vi "Get Callers Cache.vi"(8 "error in (no error)":errorcluster, 11 "WorkSpace / Repo path":path) -> (0 "error out":errorcluster, 1 "LV Version Mismatched VI":path[](array[path]), 2 "Status":string, 3 "Caller Map":map{string, string[]}(c390))   [LabVIEW 2019, in "Hawkeye.lvlib"]
uses:
  Hawkeye.lvlib
  c1dc875a-4590-4514-8f55-1f0bbeb3d42e.vi
  f2e1f123-2e97-488a-9f38-c5ab8c69dbb8.vi
  3dc4041e-3bdf-4db9-bc93-15cebc6804b8.vi
  <userlib>/_OpenG.lib/array/array.llb/Search 1D Array (String)__ogtk.vi
panel:
  # "Generating Linker Cache file"
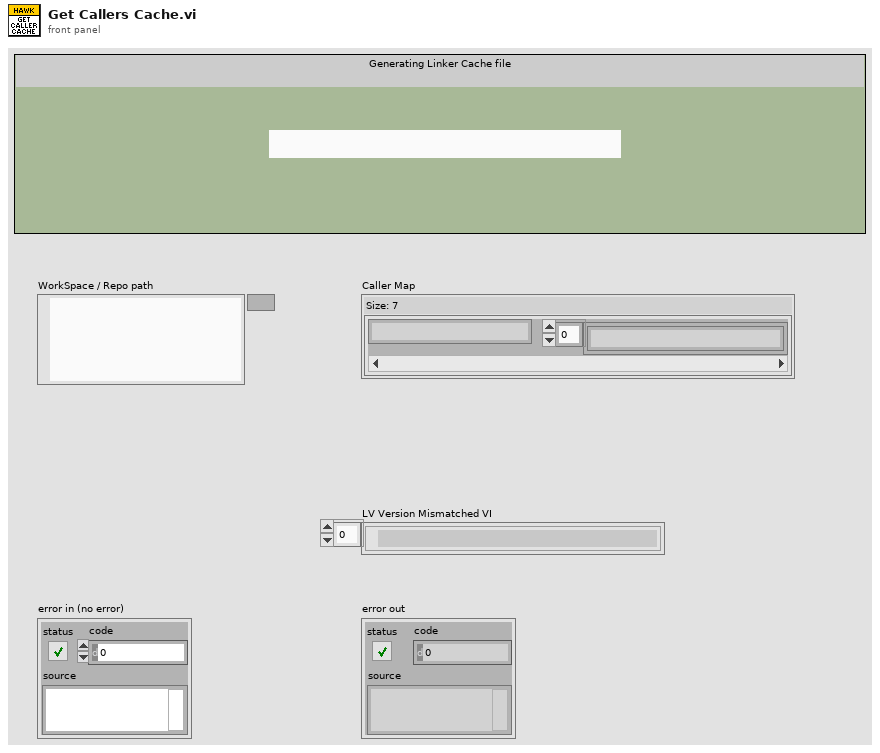
[diagram p1: front panel]
types:
  T1 = enum16{"open", "replace", "create", "open or create", "replace or create", "replace or create with confirmation"}
  T2 = typedef "NI_FileType.lvlib/LVFileType.ctl" = enum32{"Invalid file", "Unknown type", "Instrument", "Control", "Polymorphic VI", "Project", "Library", "LVClass", "XControl", "XNode", "Shared library", ".NET assembly", "ActiveX interface", "CIN", "Run-time menu", "Palette menu", "Help file", "LLB", "XNode Edit Dependency", "Class Private Data Control", "Statechart", "MathScript .m file", "Ladder Diagram", "LVLibp", "XNode Build Dependency"}
  T3 = cluster{"path":path, "delimited name":string, "type":T2, "iState":u32, "iStyle":u16, "wStyle":u16, "buttons":u16, "viflags":u32, "viflags2":u32, "links":u32[]}[]
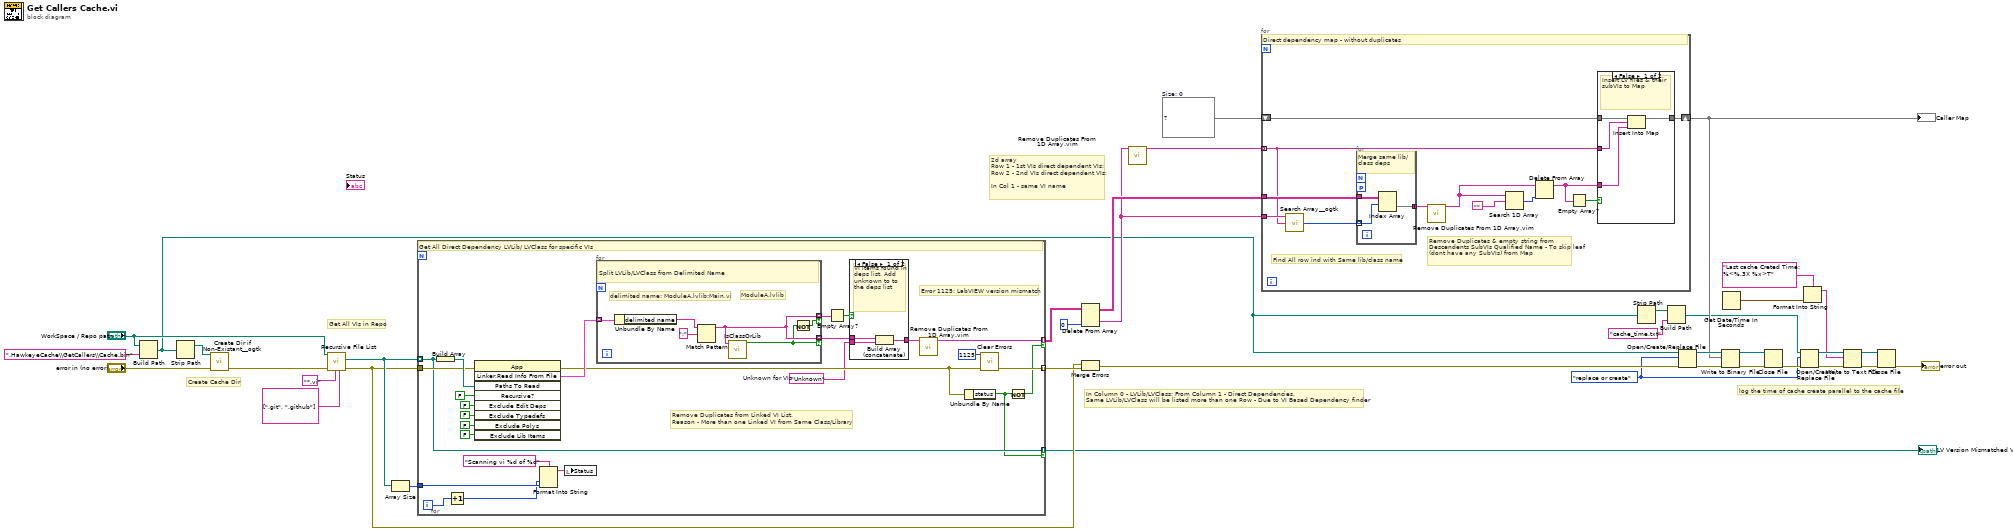
[diagram p0: block diagram]
diagram:
  w4 = T1."replace or create" ("operation (0:open)")
  w21 = map{string, string[]} {}  # Size: 0
  # "log the time of cache create parallel to the cache file"
  # "2d array \nRow 1 - 1st VIs direct dependent VIs; \nRow 2 - 2nd VIs direct dependent VIs;\n\nIn Col 1 - same VI name"
  # "In Column 0 - LVLib/LVClass; From Column 1 - Direct Dependencies.\nSame LVLib/LVClass will be listed more than one Row - Due to VI Based Dependency finder"
  # "Get All VIs in Repo"
  # "Create Cache Dir"
  n1 = Build Path(base path="WorkSpace / Repo path", name or relative path=".HawkeyeCache\\GetCallers\\Cache.bin") -> (appended path=w8:path)
  n2 = Strip Path(path=w8) -> (stripped path=w36:path)  [unwired: 1 out]
  n3 = call <userlib>:"Create Dir if Non-Existant__ogtk.vi"("error in (no error)"="error in (no error)", "Directory Path"=w36) -> ("error out"=w34:errorcluster)  [unwired: 7 in, 2 out]
  n4 = call <vilib>:"Recursive File List.vi"("Folders to Exclude"=string[] [".git", ".github"], "pattern"="*.vi", "error in (no error)"=w34, "Folder Path"="WorkSpace / Repo path") -> ("error out"=w17:errorcluster, "All Files in Dir"=w26:path[])  [unwired: 3 in, 3 out]
  n5 = Array Size(array=w26) -> (size(s)=w31:i32)
  n6 = for {
    tunnel: w31 -> [w60]
    tunnel: [w54] -> w24 mode=indexing if=w47
    tunnel: w17 -> [w56]
    tunnel: w26 -> [w50] mode=indexing
    tunnel: [w52] -> w19 mode=indexing
    tunnel: [w50] -> w15 mode=indexing if=w48
    i -> [w61]
    w43 = "Unknown"  # Unknown for VIs
    # "Error 1125: LabVIEW version mismatch"
    # "Remove Duplicates from Linked VI List.\nReason - More than one Linked VI from Same Class/Library"
    # "Get All Direct Dependency LVLib/ LVClass for specific VIs"
    n7 = Build Array(w50) -> (w62:path[])
    n8 = Increment(x=w61) -> (x+1=w57:i32)
    n9 = invoke on="Invoke Node" class="App" method="Linker.Read Info From File"(error in=w56, "Paths To Read"=w62, "Recursive?"=FALSE, "Exclude Edit Deps"=FALSE ("Exclude Edit Time Dependencies"), "Exclude Typedefs"=FALSE, "Exclude Polys"=FALSE ("Exclude Poly VIs"), "Exclude Lib Items"=FALSE ("Exclude Unused Library Items")) -> (error out=w49:errorcluster, "Linker.Read Info From File"=w55:T3)  [unwired: 2 in, 7 out]
    n10 = Format Into String(format string="Scanning vi %d of %d", w57, w60) -> (resulting string=w58:string)  [unwired: 2 in, 1 out]
    n11 = local write "Status"(w58) -> ()
    n12 = for {
      tunnel: w55 -> [w73] mode=indexing
      tunnel: [w70] -> w53 mode=indexing if=w69
      tunnel: [w70] -> w44 mode=indexing if=w68
      # "ModuleA.lvlib"
      # "delimited name: ModuleA.lvlib:Main.vi"
      # "Split LVLib/LVClass from Delimited Name"
      n13 = Unbundle By Name(w73) -> ("delimited name"=w71:string)
      n14 = Match Pattern(string=w71, regular expression=":") -> (before substring=w70:string)  [unwired: 1 in, 3 out]
      n15 = call "IsClassOrLib.vi"("LVFile Name"=w70) -> ("Is LVClass or Library?"=w69:bool)  [unwired: 9 in, 1 out]
      n16 = Not(x=w69) -> (.not. x?=w68:bool)
    }
    n17 = Empty Array?(array=w44) -> (empty?=w46:bool)
    n18 = case shown="False" w46 {
      tunnel: w53 -> [w66 w67]
      tunnel: [w65 w67] -> w45
      tunnel: w43 -> [w64 _]
      frame False {
        # "VI items found in deps list. Add unknown to to the deps list"
        n19 = Build Array (concatenate)(w66, w64) -> (w65:string[])
      }
      frame True {
        # "Only class & lib in deps list"
      }
    }
    n20 = call "Remove Duplicates From 1D Array.vim"("array"=w45) -> ("array with duplicates removed"=w54:string[])  [unwired: 10 in]
    n21 = Unbundle By Name(w49) -> ("status"=w48:bool)
    n22 = call <vilib>:"Clear Errors.vi"("error in (no error)"=w49, "specific error code to clear (0: all)"=1125) -> ("error out"=w52:errorcluster)  [unwired: 4 in, 1 out]
    n23 = Not(x=w48) -> (.not. x?=w47:bool)
  }
  "LV Version Mismatched VI" <- w15
  n24 = Merge Errors(w17, w19) -> (w18:errorcluster)
  n25 = Delete From Array(array=w24, index (col)=0 ("disabled index (col)")) -> (deleted portion=w22:string[], array with subset deleted=w23:string[][])  [unwired: 2 in]
  n26 = call "Remove Duplicates From 1D Array.vim"("array"=w22) -> ("array with duplicates removed"=w16:string[])  [unwired: 10 in]
  n27 = for {
    tunnel: w16 -> [w81] mode=indexing
    tunnel: w22 -> [w85]
    shift-right: [w82] -> w20
    shift-left: w21 -> [w84]
    tunnel: w23 -> [w83]
    # "Find All row ind with Same lib/class name"
    # "Remove Duplicates & empty string from \nDescendents SubVIs Qualified Name - To skip leaf (dont have any SubVIs) from Map"
    # "Direct dependency map - without duplicates"
    n28 = call-poly <userlib>:"Search Array__ogtk.vi"("Array"=w85, "Element Data"=w81) -> ("Indices of Elements"=w75:i32[])  [unwired: 7 in]
    n29 = for {
      tunnel: w83 -> [w88]
      tunnel: w75 -> [w87] mode=indexing
      tunnel: [w86] -> w74 mode=concatenating
      workers-P: _ -> [_]
      # "Merge same lib/class deps"
      n30 = Index Array(array=w88, index (row)=w87) -> (element=w86:string[])  [unwired: 1 in]
    }
    n31 = call "Remove Duplicates From 1D Array.vim"("array"=w74) -> ("array with duplicates removed"=w78:string[])  [unwired: 10 in]
    n32 = Search 1D Array(1D array=w78, element="" ("Empty String Constant")) -> (index of element=w79:i32)  [unwired: 1 in]
    n33 = Delete From Array(array=w78, index=w79) -> (array with subset deleted=w76:string[])  [unwired: 1 in, 1 out]
    n34 = Empty Array?(array=w76) -> (empty?=w77:bool)
    n35 = case shown="False" w77 {
      tunnel: [w92 w93] -> w82
      tunnel: w84 -> [w91 w93]
      tunnel: w81 -> [w89 _]
      tunnel: w76 -> [w90 _]
      frame False {
        # "Insert LV files & their subVIs to Map"
        n36 = Insert Into Map(map in=w91, key=w89, value=w90) -> (map out=w92:map{string, string[]})  [unwired: 2 out]
      }
      frame True {
      }
    }
  }
  "Caller Map" <- w20
  n37 = Strip Path(path=w8) -> (stripped path=w10:path)  [unwired: 1 out]
  n38 = Build Path(base path=w10, name or relative path="cache_time.txt") -> (appended path=w7:path)
  n39 = Open/Create/Replace File(file path (use dialog)=w8, error in=w18, operation (0:open)=w4) -> (refnum out=w30:refnum<file>, error out=w27:errorcluster)  [unwired: 3 in, 1 out]
  n40 = Write to Binary File(file (use dialog)=w30, data=w20, error in=w27) -> (refnum out=w29:refnum<file>, error out=w28:errorcluster)  [unwired: 3 in, 1 out]
  n41 = Get Date/Time In Seconds() -> (seconds since 1Jan1904=w2:timestamp)
  n42 = Close File(refnum=w29, error in=w28) -> (error out=w6:errorcluster)  [unwired: 1 out]
  n43 = Open/Create/Replace File(file path (use dialog)=w7, error in=w6, operation (0:open)=w4) -> (refnum out=w12:refnum<file>, error out=w14:errorcluster)  [unwired: 3 in, 1 out]
  n44 = Format Into String(format string="Last cache Creted Time: %<%.3X %x>T" ("name or relative path"), w2) -> (resulting string=w1:string)  [unwired: 2 in, 1 out]
  n45 = Write to Text File(file (use dialog)=w12, text=w1, error in=w14) -> (refnum out=w11:refnum<file>, error out=w13:errorcluster)  [unwired: 1 in, 1 out]
  n46 = Close File(refnum=w11, error in=w13) -> (error out=→"error out":errorcluster)  [unwired: 1 out]
